vi "ApplicationConfigWriteIniFile.vi"(8 "error in (no error)":errorcluster, 10 "IniFilePath":path, 11 "ApplicationConfig":T1) -> (0 "error out":errorcluster)   [LabVIEW 2013]
uses:
  Ctrls/ApplicationConfig.ctl
  Ctrls/MessageHandlerConfig.ctl
  EnumApplicationConfigIniKeys.ctl
  EnumApplicationConfigIniSections.ctl
  <vilib>/Utility/config.llb/Write Key (Path).vi
  <vilib>/Utility/config.llb/Write Key (Boolean).vi
  <vilib>/Utility/config.llb/Write Key (U32).vi
  <vilib>/Utility/config.llb/Write Key (String).vi
  <vilib>/Utility/config.llb/NI_LVConfig.lvlib
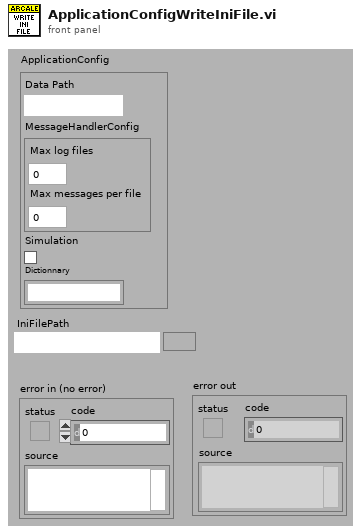
[diagram p1: front panel]
types:
  T1 = typedef "ApplicationConfig.ctl" = cluster{"Data Path":path, "MessageHandlerConfig":T2, "Simulation":bool, "Dictionnary":string}
  T2 = typedef "MessageHandlerConfig.ctl" = cluster{"Max log files":u32, "Max messages per file":u32}
  T3 = typedef "EnumApplicationConfigIniKeys.ctl" = enum16{"Simulation", "Data path", "Max LOG files", "Max message per LOG file", "Dictionnary"}
  T4 = typedef "EnumApplicationConfigIniSections.ctl" = enum16{"GLOBAL", "LOG", "LOCALIZATION"}
  T5 = typedef "NI_LVConfig.lvlib/Config Data RefNum.ctl" = refnum<k1>
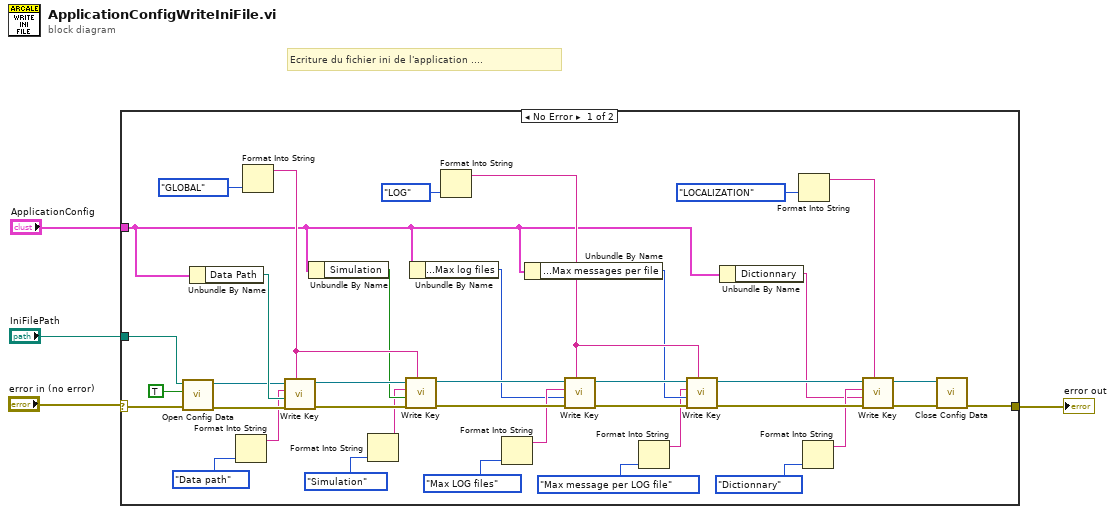
[diagram p0: block diagram]
diagram:
  # "Ecriture du fichier ini de l'application ...."
  n1 = case shown="No Error" "error in (no error)" {
    selector: "error in (no error)" -> [w42 w43]
    tunnel: [w18 w43] -> w3
    tunnel: "IniFilePath" -> [w41 _]
    tunnel: "ApplicationConfig" -> [w6 _]
    frame No Error {
      n2 = call <vilib>:"Open Config Data.vi"("error in (no error)"=w42, "create file if necessary (T)"=TRUE, "configuration file path"=w41) -> ("error out"=w39:errorcluster, "refnum"=w37:T5)  [unwired: 6 in, 1 out]
      n3 = Unbundle By Name(w6) -> ("Data Path"=w38:path)
      n4 = Format Into String(EnumApplicationConfigIniKeys."Data path" ("Clé")) -> (resulting string=w34:string)  [unwired: 3 in, 1 out]
      n5 = Format Into String(EnumApplicationConfigIniSections."GLOBAL" ("Section")) -> (resulting string=w31:string)  [unwired: 3 in, 1 out]
      n6 = call-poly <vilib>:"Write Key.vi"("section"=w31, "error in (no error)"=w39, "value"=w38, "key"=w34, "refnum"=w37) -> ("error out"=w33:errorcluster, "refnum out"=w32:T5)  [unwired: 4 in, 1 out]
      n7 = Unbundle By Name(w6) -> ("Simulation"=w30:bool)
      n8 = Format Into String(EnumApplicationConfigIniKeys."Simulation" ("Clé")) -> (resulting string=w28:string)  [unwired: 3 in, 1 out]
      n9 = call-poly <vilib>:"Write Key.vi"("section"=w31, "error in (no error)"=w33, "value"=w30, "key"=w28, "refnum"=w32) -> ("error out"=w26:errorcluster, "refnum out"=w25:T5)  [unwired: 4 in, 1 out]
      n10 = Unbundle By Name(w6) -> ("MessageHandlerConfig.Max log files"=w22:u32)
      n11 = Format Into String(EnumApplicationConfigIniSections."LOG" ("Section")) -> (resulting string=w19:string)  [unwired: 3 in, 1 out]
      n12 = Format Into String(EnumApplicationConfigIniKeys."Max LOG files" ("Clé")) -> (resulting string=w23:string)  [unwired: 3 in, 1 out]
      n13 = Unbundle By Name(w6) -> ("MessageHandlerConfig.Max messages per file"=w17:u32)
      n14 = call-poly <vilib>:"Write Key.vi"("section"=w19, "error in (no error)"=w26, "value"=w22, "key"=w23, "refnum"=w25) -> ("error out"=w21:errorcluster, "refnum out"=w20:T5)  [unwired: 4 in, 1 out]
      n15 = Format Into String(EnumApplicationConfigIniKeys."Max message per LOG file" ("Clé")) -> (resulting string=w15:string)  [unwired: 3 in, 1 out]
      n16 = call-poly <vilib>:"Write Key.vi"("section"=w19, "error in (no error)"=w21, "value"=w17, "key"=w15, "refnum"=w20) -> ("error out"=w12:errorcluster, "refnum out"=w14:T5)  [unwired: 4 in, 1 out]
      n17 = Unbundle By Name(w6) -> ("Dictionnary"=w5:string)
      n18 = Format Into String(EnumApplicationConfigIniSections."LOCALIZATION" ("Section")) -> (resulting string=w9:string)  [unwired: 3 in, 1 out]
      n19 = Format Into String(EnumApplicationConfigIniKeys."Dictionnary" ("Clé")) -> (resulting string=w7:string)  [unwired: 3 in, 1 out]
      n20 = call-poly <vilib>:"Write Key.vi"("section"=w9, "error in (no error)"=w12, "value"=w5, "key"=w7, "refnum"=w14) -> ("error out"=w11:errorcluster, "refnum out"=w13:T5)  [unwired: 4 in, 1 out]
      n21 = call <vilib>:"Close Config Data.vi"("error in (no error)"=w11, "refnum"=w13) -> ("error out"=w18:errorcluster)  [unwired: 8 in, 1 out]
    }
    frame Error {
    }
  }
  "error out" <- w3
